vi "诊断标定3.vi"(8 "CAN端口":u16(ring), 9 "设备索引号":u16(ring), 10 "CAN卡类型":u32(ring)=21) -> ()   [LabVIEW 2013] (continued)
                      tunnel: [_ u8 128 ("命令") u8 129 ("命令") u8 128 ("命令") u8 140 ("命令") u8 128 ("命令") u8 128 ("命令") u8 128 ("命令") u8 128 ("命令") u8 128 ("命令") u8 128 ("命令") u8 128 ("命令") u8 128 ("命令") u8 128 ("命令") u8 128 ("命令") u8 128 ("命令") u8 128 ("命令") u8 128 ("命令") u8 129 ("命令") u8 129 ("命令") u8 130 ("命令") u8 130 ("命令") u8 132 ("命令") u8 132 ("命令") u8 132 ("命令") u8 132 ("命令") u8 132 ("命令")] -> w4352
                      tunnel: [_ string[] ["产品编号", "电压个数", "通道电压数", "电压起始值", "温度个数", "温度起始值", "保险位置", "电池额定实际容量", "SOC", "配置文件版本", "参数修改记录", "车牌号", "SOH"] string[] ["一级故障阀值"] string[] ["产品编号"] string[] ["读二维码"] string[] ["电压个数"] string[] ["通道电压数"] string[] ["电压起始值"] string[] ["温度个数"] string[] ["温度起始值"] string[] ["保险位置"] string[] ["SOC"] string[] ["电池额定实际容量"] string[] ["配置文件版本"] string[] ["参数修改记录"] string[] ["校正时钟"] string[] ["车牌号"] string[] ["SOH"] string[] ["二级故障阀值"] string[] ["三级故障阀值"] string[] ["加热控制参数"] string[] ["充电控制参数"] string[] ["电池信息1"] string[] ["电池包组号"] string[] ["充放电安时"] string[] ["电池充放电次数"] string[] ["电池信息1", "电池包组号", "充放电安时", "电池充放电次数"]] -> w4348
                      frame "假", Default {
                      }
                      frame "项目信息" {
                      }
                      frame "SOC过低", "SOC过高", "SOH过低", "充电电流过高", "单体电压过低", "单体电压过高", "单组电压不均衡", "单组温度不均衡", "放电电流过高", "极柱温度过高", "内阻过大", "温度过低", "温度过高", "一级故障阀值", "整组电压不均衡", "整组温度不均衡", "总电压过低", "总电压过高" {
                      }
                      frame "产品编号" {
                      }
                      frame "二维码" {
                      }
                      frame "电压个数" {
                      }
                      frame "通道电压数" {
                      }
                      frame "电压起始值" {
                      }
                      frame "温度个数" {
                      }
                      frame "温度起始值" {
                      }
                      frame "保险位置" {
                      }
                      frame "SOC" {
                      }
                      frame "电池额定实际容量" {
                      }
                      frame "配置文件版本" {
                      }
                      frame "参数修改记录" {
                      }
                      frame "校正时钟" {
                      }
                      frame "车牌号" {
                      }
                      frame "SOH" {
                      }
                      frame "SOC过低(2)", "SOC过高(2)", "SOH过低(2)", "充电电流过高(2)", "单体电压过低(2)", "单体电压过高(2)", "单组电压不均衡(2)", "单组温度不均衡(2)", "二级故障阀值", "放电电流过高(2)", "极柱温度过高(2)", "内阻过大(2)", "温度过低(2)", "温度过高(2)", "整组电压不均衡(2)", "整组温度不均衡(2)", "总电压过低(2)", "总电压过高(2)" {
                      }
                      frame "SOC过低(3)", "SOC过高(3)", "SOH过低(3)", "充电电流过高(3)", "单体电压过低(3)", "单体电压过高(3)", "单组电压不均衡(3)", "单组温度不均衡(3)", "放电电流过高(3)", "极柱温度过高(3)", "内阻过大(3)", "三级故障阀值", "温度过低(3)", "温度过高(3)", "整组电压不均衡(3)", "整组温度不均衡(3)", "总电压过低(3)", "总电压过高(3)" {
                      }
                      frame "风机关闭温差", "风机关闭温度", "风机开启温差", "风机开启温度", "加热关闭温差", "加热关闭温度", "加热开启温度", "加热控制参数" {
                      }
                      frame "充电控制参数", "电流步长", "最大允许充电电流", "最大允许充电温度", "最大允许单体电压", "最大允许总电压", "最小允许充电电流", "最小允许充电温度", "最小允许单体电压" {
                      }
                      frame "电池信息1" {
                      }
                      frame "电池包组号" {
                      }
                      frame "充放电安时" {
                      }
                      frame "电池充放电次数" {
                      }
                      frame "电池信息" {
                      }
                    }
                  }
                  frame "从板" {
                    n3274 = local read "从板选项"() -> (w4434:string)
                    n3275 = case shown="\"二维码\"" w4434 {
                      tunnel: [_ u8 0 ("命令") u8 10 ("命令") u8 0 ("命令") u8 0 ("命令") u8 0 ("命令") u8 0 ("命令") u8 0 ("命令") u8 0 ("命令") u8 2 ("命令") u8 2 ("命令") u8 2 ("命令") u8 3 ("命令") u8 6 ("命令") u8 6 ("命令") u8 6 ("命令") u8 3 ("命令") u8 3 ("命令") u8 3 ("命令") u8 3 ("命令") u8 3 ("命令") u8 3 ("命令") u8 3 ("命令")] -> w4437
                      tunnel: [_ u8[] [6] u8[] [1] u8[] [6, 1, 2, 3, 4, 5] u8[] [1] u8[] [2] u8[] [3] u8[] [4] u8[] [5] u8[] [1] u8[] [2] u8[] [3] u8[] [1, 2, 3, 4, 5, 6, 7] u8[] [1, 2] u8[] [2] u8[] [1] u8[] [1] u8[] [2] u8[] [3] u8[] [4] u8[] [5] u8[] [6] u8[] [7]] -> w4436
                      tunnel: [_ string[] ["从板号"] string[] ["读二维码"] string[] ["从板号", "电压起始值", "通道电压个数", "保险位置", "温度起始值", "加热控制参数"] string[] ["电压起始值"] string[] ["通道电压节数"] string[] ["保险位置"] string[] ["温度起始值"] string[] ["加热控制参数"] string[] ["一级故障阀值"] string[] ["二级故障阀值"] string[] ["三级故障阀值"] string[] ["电池包信息1", "电池包序号", "充放电安时", "充电次数时间", "SOC", "车牌号", "充电参数"] string[] ["均衡阀值", "充电结束电压"] string[] ["充电结束电压"] string[] ["均衡阀值"] string[] ["电池包信息1"] string[] ["电池包序号"] string[] ["充放电安时"] string[] ["充电次数时间"] string[] ["SOC"] string[] ["车牌号"] string[] ["充电参数"]] -> w4432
                      frame "假", Default {
                      }
                      frame "从板号" {
                      }
                      frame "二维码" {
                      }
                      frame "从板信息" {
                      }
                      frame "电压个数" {
                      }
                      frame "通道电压节数" {
                      }
                      frame "保险位置" {
                      }
                      frame "温度个数" {
                      }
                      frame "风机关闭温差", "风机关闭温度", "风机开启温差", "风机开启温度", "加热关闭温差", "加热关闭温度", "加热开启温度", "加热控制参数" {
                      }
                      frame "SOC过低", "电压不均衡", "电压过低", "电压过高", "温度不均衡", "温度过低", "温度过高", "一级故障阀值" {
                      }
                      frame "SOC过低(2)", "电压不均衡(2)", "电压过低(2)", "电压过高(2)", "二级故障阀值", "温度不均衡(2)", "温度过低(2)", "温度过高(2)" {
                      }
                      frame "SOC过低(3)", "电压不均衡(3)", "电压过低(3)", "电压过高(3)", "三级故障阀值", "温度不均衡(3)", "温度过低(3)", "温度过高(3)" {
                      }
                      frame "快换参数" {
                      }
                      frame "均衡参数" {
                      }
                      frame "充电结束电压" {
                      }
                      frame "均衡阀值" {
                      }
                      frame "电池包信息1" {
                      }
                      frame "电池包序号" {
                      }
                      frame "充放电安时" {
                      }
                      frame "充电次数时间" {
                      }
                      frame "SOC" {
                      }
                      frame "车牌号" {
                      }
                      frame "充电参数" {
                      }
                    }
                    n3276 = local read "从板号"() -> (w4433:u8)
                  }
                }
                n3277 = Build Array(w4345) -> (w4344:i32[])
                n3278 = local write "命令"(w4347) -> ()
                n3279 = Array Size(array=w4342) -> (size(s)=w4341:i32)
                n3280 = for {
                  tunnel: w4342 -> [w4512] mode=indexing
                  tunnel: w4347 -> [w4511]
                  tunnel: w4346 -> [w4510]
                  tunnel: w4344 -> [w4509]
                  tunnel: w4343 -> [w4508] mode=indexing
                  tunnel: w4341 -> [w4507]
                  tunnel: w4340 -> [w4505]
                  tunnel: [w4504] -> w4339
                  i -> [w4506]
                  n3281 = while {
                    tunnel: w4512 -> [w4521]
                    tunnel: w4511 -> [w4520]
                    tunnel: w4510 -> [w4519]
                    tunnel: w4509 -> [w4518]
                    tunnel: w4508 -> [w4517]
                    tunnel: w4507 -> [w4516]
                    tunnel: w4506 -> [w4515]
                    tunnel: w4505 -> [w4514]
                    tunnel: [w4513] -> w4504
                    stop <- w4513 stop-if-true
                    n3282 = stacked-sequence {
                      seq-local: [_ _ _ _ w4671 _ _] -> [_ _ _ _ _ w4680 _]
                      tunnel: w4521 -> [_ _ _ w4659 _ _ _]
                      tunnel: w4520 -> [_ _ _ w4658 _ _ _]
                      tunnel: w4519 -> [_ _ _ w4657 _ _ _]
                      tunnel: w4518 -> [_ _ _ w4656 _ _ _]
                      tunnel: [_ _ _ _ w4672 _ _] -> w4513
                      tunnel: w4517 -> [w4523 _ _ _ _ w4681 _]
                      tunnel: w4516 -> [_ _ _ _ _ _ w4691]
                      tunnel: w4515 -> [_ _ _ _ _ _ w4690]
                      tunnel: w4514 -> [w4522 _ _ _ _ _ _]
                      frame #0 {
                        n3283 = case shown="\"从板\"" w4522 {
                          tunnel: w4523 -> [w4524 w4616]
                          frame "主板", Default {
                            n3284 = case shown="\"读二维码\"" w4524 {
                              frame "假", Default {
                              }
                              frame "产品编号" {
                                n3285 = control-ref of="产品编号"() -> (w4526:refnum<vi>)
                                n3286 = property class="Str"(reference=w4526, "Value"="") -> ()  [unwired: 1 in, 2 out]
                              }
                              frame "读二维码" {
                                n3287 = local write "二维码信息"("" ("二维码信息")) -> ()
                              }
                              frame "电压个数" {
                                n3288 = local read "从板个数"() -> (w4528:dbl)
                                n3289 = control-ref of="项目信息"() -> (w4532:refnum<vi>)
                                n3290 = for {
                                N: w4528 -> [_]
                                tunnel: [""] -> w4531 mode=indexing
                                }
                                n3291 = call "表格数据输入-8.6.vi"("行数"=u32 0, "列数"=u32 1, "字符串数组"=w4531, "表格引用"=w4532) -> ()  [unwired: 8 in]
                              }
                              frame "通道电压数" {
                                n3292 = control-ref of="项目信息"() -> (w4538:refnum<vi>)
                                n3293 = for {
                                N: 20 -> [_]
                                tunnel: [""] -> w4537 mode=indexing
                                }
                                n3294 = local read "从板个数"() -> (w4539:dbl)
                                n3295 = Increment(x=w4539) -> (x+1=w4535:dbl)
                                n3296 = call "表格数据输入-8.6.vi"("行数"=w4535, "列数"=u32 1, "字符串数组"=w4537, "表格引用"=w4538) -> ()  [unwired: 8 in]
                              }
                              frame "电压起始值" {
                                n3297 = local read "从板个数"() -> (w4543:dbl)
                                n3298 = Increment(x=w4543) -> (x+1=w4542:dbl)
                                n3299 = control-ref of="项目信息"() -> (w4549:refnum<vi>)
                                n3300 = for {
                                N: w4542 -> [_]
                                tunnel: [""] -> w4548 mode=indexing
                                }
                                n3301 = Multiply(x=u8 1, y=w4543) -> (x*y=w4545:dbl)
                                n3302 = Add(x=w4545, y=u8 21) -> (x+y=w4541:dbl)
                                n3303 = call "表格数据输入-8.6.vi"("行数"=w4541, "列数"=u32 1, "字符串数组"=w4548, "表格引用"=w4549) -> ()  [unwired: 8 in]
                              }
                              frame "温度个数" {
                                n3304 = local read "从板个数"() -> (w4553:dbl)
                                n3305 = Increment(x=w4553) -> (x+1=w4552:dbl)
                                n3306 = control-ref of="项目信息"() -> (w4559:refnum<vi>)
                                n3307 = for {
                                N: w4552 -> [_]
                                tunnel: [""] -> w4558 mode=indexing
                                }
                                n3308 = Multiply(x=u8 2, y=w4553) -> (x*y=w4555:dbl)
                                n3309 = Add(x=w4555, y=u8 22) -> (x+y=w4551:dbl)
                                n3310 = call "表格数据输入-8.6.vi"("行数"=w4551, "列数"=u32 1, "字符串数组"=w4558, "表格引用"=w4559) -> ()  [unwired: 8 in]
                              }
                              frame "温度起始值" {
                                n3311 = local read "从板个数"() -> (w4563:dbl)
                                n3312 = Increment(x=w4563) -> (x+1=w4562:dbl)
                                n3313 = control-ref of="项目信息"() -> (w4569:refnum<vi>)
                                n3314 = for {
                                N: w4562 -> [_]
                                tunnel: [""] -> w4568 mode=indexing
                                }
                                n3315 = Multiply(x=u8 3, y=w4563) -> (x*y=w4565:dbl)
                                n3316 = Add(x=w4565, y=u8 23) -> (x+y=w4561:dbl)
                                n3317 = call "表格数据输入-8.6.vi"("行数"=w4561, "列数"=u32 1, "字符串数组"=w4568, "表格引用"=w4569) -> ()  [unwired: 8 in]
                              }
                              frame "保险位置" {
                                n3318 = local read "从板个数"() -> (w4573:dbl)
                                n3319 = control-ref of="项目信息"() -> (w4579:refnum<vi>)
                                n3320 = for {
                                N: 10 -> [_]
                                tunnel: [""] -> w4578 mode=indexing
                                }
                                n3321 = Multiply(x=u8 4, y=w4573) -> (x*y=w4575:dbl)
                                n3322 = Add(x=w4575, y=u8 24) -> (x+y=w4572:dbl)
                                n3323 = call "表格数据输入-8.6.vi"("行数"=w4572, "列数"=u32 1, "字符串数组"=w4578, "表格引用"=w4579) -> ()  [unwired: 8 in]
                              }
                              frame "电池额定实际容量" {
                                w4581 = 0.0 ("值")
                                n3324 = control-ref of="电池实际容量(A)"() -> (w4582:refnum<vi>)
                                n3325 = control-ref of="电池额定容量(A)"() -> (w4583:refnum<vi>)
                                n3326 = property class="DigNum (严格)"(reference=w4582, "Value"=w4581) -> ()  [unwired: 1 in, 2 out]
                                n3327 = property class="DigNum (严格)"(reference=w4583, "Value"=w4581) -> ()  [unwired: 1 in, 2 out]
                              }
                              frame "SOC" {
                                n3328 = control-ref of="SOC(%)"() -> (w4584:refnum<vi>)
                                n3329 = property class="DigNum (严格)"(reference=w4584, "Value"=0.0 ("值")) -> ()  [unwired: 1 in, 2 out]
                              }
                              frame "配置文件版本" {
                                n3330 = control-ref of="配置文件版本"() -> (w4586:refnum<vi>)
                                n3331 = property class="Str"(reference=w4586, "Value"="" ("值")) -> ()  [unwired: 1 in, 2 out]
                              }
                              frame "参数修改记录" {
                                n3332 = control-ref of="使用者"() -> (w4589:refnum<vi>)
                                n3333 = control-ref of="系统时钟"() -> (w4590:refnum<vi>)
                                n3334 = property class="DigNum (严格)"(reference=w4589, "Value"=0.0 ("值")) -> ()  [unwired: 1 in, 2 out]
                                n3335 = property class="Str"(reference=w4590, "Value"="" ("值")) -> ()  [unwired: 1 in, 2 out]
                              }
                              frame "校正时钟" {
                                n3336 = control-ref of="系统时钟"() -> (w4592:refnum<vi>)
                                n3337 = property class="Str"(reference=w4592, "Value"="" ("值")) -> ()  [unwired: 1 in, 2 out]
                              }
                              frame "车牌号" {
                                n3338 = control-ref of="车架(牌)号"() -> (w4594:refnum<vi>)
                                n3339 = property class="Str"(reference=w4594, "Value"="" ("值")) -> ()  [unwired: 1 in, 2 out]
                              }
                              frame "SOH" {
                                n3340 = control-ref of="SOH(%)"() -> (w4597:refnum<vi>)
                                n3341 = property class="DigNum (严格)"(reference=w4597, "Value"=0.0 ("值")) -> ()  [unwired: 1 in, 2 out]
                              }
                              frame "一级故障阀值" {
                                n3342 = local write "一级故障"(T10 {"总电压过高"=0.0, "整组电压不均衡"=0.0, "SOC过高"=0.0, "单体电压过高"=0.0, "总电压过低"=0.0, "温度过高"=0.0, "温度过低"=0.0, "单组电压不均衡"=0.0, "整组温度不均衡"=0.0, "单组温度不均衡"=0.0, "单体电压过低"=0.0, "充电电流过高"=0.0, "放电电流过高"=0.0, "SOC过低"=0.0, "内阻过大"=0.0, "极柱温度过高"=0.0, "SOH过低"=0.0} ("一级故障")) -> ()
                              }
                              frame "二级故障阀值" {
                                n3343 = local write "一级故障 2"(T10 {"总电压过高"=0.0, "整组电压不均衡"=0.0, "SOC过高"=0.0, "单体电压过高"=0.0, "总电压过低"=0.0, "温度过高"=0.0, "温度过低"=0.0, "单组电压不均衡"=0.0, "整组温度不均衡"=0.0, "单组温度不均衡"=0.0, "单体电压过低"=0.0, "充电电流过高"=0.0, "放电电流过高"=0.0, "SOC过低"=0.0, "内阻过大"=0.0, "极柱温度过高"=0.0, "SOH过低"=0.0} ("一级故障")) -> ()
                              }
                              frame "三级故障阀值" {
                                n3344 = local write "一级故障 3"(T10 {"总电压过高"=0.0, "整组电压不均衡"=0.0, "SOC过高"=0.0, "单体电压过高"=0.0, "总电压过低"=0.0, "温度过高"=0.0, "温度过低"=0.0, "单组电压不均衡"=0.0, "整组温度不均衡"=0.0, "单组温度不均衡"=0.0, "单体电压过低"=0.0, "充电电流过高"=0.0, "放电电流过高"=0.0, "SOC过低"=0.0, "内阻过大"=0.0, "极柱温度过高"=0.0, "SOH过低"=0.0} ("一级故障")) -> ()
                              }
                              frame "加热控制参数" {
                                n3345 = local write "加热控制参数"(T11 {"风机开启温度"=0.0, "风机关闭温度"=0.0, "加热开启温度"=0.0, "加热关闭温度"=0.0, "风机开启温差"=0.0, "风机关闭温差"=0.0, "加热关闭温差"=0.0} ("加热控制参数")) -> ()
                              }
                              frame "充电控制参数" {
                                n3346 = local write "一级故障 5"(T12 {"最大允许单体电压"=0.0, "最大允许总电压"=0.0, "最小允许单体电压"=0.0, "最大允许充电电流"=0.0, "最小允许充电电流"=0.0, "最大允许充电温度"=0.0, "最小允许充电温度"=0.0, "电流步长"=0.0} ("一级故障 5")) -> ()
                              }
                              frame "电池信息1" {
                                w4603 = ""
                                w4604 = 0.0 ("电池串联")
                                n3347 = local read "电池信息"() -> (w4606:T13)
                                n3348 = Bundle By Name(cluster=w4606, "电池串联"=w4604, "电池并联"=w4604, "电池包额定容量"=w4604, "电池包额定能量(kWh)"=w4604, "电池包额定总电压"=w4604, "实际容量"=w4604, "电池厂家"=w4603, "电池类型"=w4603, "电池生产日期"=w4603) -> (w4605:T13)
                                n3349 = local write "电池信息"(w4605) -> ()
                              }
                              frame "电池包组号" {
                                n3350 = local read "电池信息"() -> (w4609:T13)
                                n3351 = Bundle By Name(cluster=w4609, "电池包组号"="") -> (w4608:T13)
                                n3352 = local write "电池信息"(w4608) -> ()
                              }
                              frame "充放电安时" {
                                w4610 = 0.0 ("累计充电总安时")
                                n3353 = local read "电池信息"() -> (w4612:T13)
                                n3354 = Bundle By Name(cluster=w4612, "累计充电总安时"=w4610, "累计放电总安时"=w4610) -> (w4611:T13)
                                n3355 = local write "电池信息"(w4611) -> ()
                              }
                              frame "电池充放电次数" {
                                w4613 = 0.0 ("累计充电总安时")
                                n3356 = local read "电池信息"() -> (w4615:T13)
                                n3357 = Bundle By Name(cluster=w4615, "电池充满次数"=w4613, "电池放空次数"=w4613, "电池充电次数"=w4613) -> (w4614:T13)
                                n3358 = local write "电池信息"(w4614) -> ()
                              }
                            }
                          }
                          frame "从板" {
                            n3359 = case shown="\"读二维码\"" w4616 {
                              frame "假", Default {
                              }
                              frame "电压起始值" {
                                n3360 = control-ref of="项目信息 2"() -> (w4618:refnum<vi>)
                                n3361 = for {
                                N: 1 -> [_]
                                tunnel: [""] -> w4621 mode=indexing
                                }
                                n3362 = call "表格数据输入-8.6.vi"("行数"=u32 0, "列数"=u32 1, "字符串数组"=w4621, "表格引用"=w4618) -> ()  [unwired: 8 in]
                              }
                              frame "读二维码" {
                                n3363 = local write "二维码信息 2"("" ("二维码信息 2")) -> ()
                              }
                              frame "通道电压节数" {
                                n3364 = control-ref of="项目信息 2"() -> (w4624:refnum<vi>)
                                n3365 = for {
                                N: 5 -> [_]
                                tunnel: [""] -> w4628 mode=indexing
                                }
                                n3366 = call "表格数据输入-8.6.vi"("行数"=u32 22, "列数"=u32 1, "字符串数组"=w4628, "表格引用"=w4624) -> ()  [unwired: 8 in]
                              }
                              frame "保险位置" {
                                n3367 = control-ref of="项目信息 2"() -> (w4630:refnum<vi>)
                                n3368 = for {
                                N: 20 -> [_]
                                tunnel: [""] -> w4634 mode=indexing
                                }
                                n3369 = call "表格数据输入-8.6.vi"("行数"=u32 2, "列数"=u32 1, "字符串数组"=w4634, "表格引用"=w4630) -> ()  [unwired: 8 in]
                              }
                              frame "温度起始值" {
                                n3370 = control-ref of="项目信息 2"() -> (w4636:refnum<vi>)
                                n3371 = for {
                                N: 1 -> [_]
                                tunnel: [""] -> w4640 mode=indexing
                                }
                                n3372 = call "表格数据输入-8.6.vi"("行数"=u32 1, "列数"=u32 1, "字符串数组"=w4640, "表格引用"=w4636) -> ()  [unwired: 8 in]
                              }
                              frame "加热控制参数" {
                                n3373 = local write "加热控制参数"(T11 {"风机开启温度"=0.0, "风机关闭温度"=0.0, "加热开启温度"=0.0, "加热关闭温度"=0.0, "风机开启温差"=0.0, "风机关闭温差"=0.0, "加热关闭温差"=0.0} ("加热控制参数")) -> ()
                              }
                              frame "一级故障阀值" {
                                n3374 = local write "一级故障 6"(T15 {"电压过高"=0.0, "电压过低"=0.0, "温度过高"=0.0, "温度过低"=0.0, "电压不均衡(V)"=0.0, "温度不均衡"=0.0, "SOC过低"=0.0} ("一级故障 6")) -> ()
                              }
                              frame "二级故障阀值" {
                                n3375 = local write "一级故障 7"(T15 {"电压过高"=0.0, "电压过低"=0.0, "温度过高"=0.0, "温度过低"=0.0, "电压不均衡(V)"=0.0, "温度不均衡"=0.0, "SOC过低"=0.0} ("一级故障 7")) -> ()
                              }
                              frame "三级故障阀值" {
                                n3376 = local write "一级故障 8"(T15 {"电压过高"=0.0, "电压过低"=0.0, "温度过高"=0.0, "温度过低"=0.0, "电压不均衡(V)"=0.0, "温度不均衡"=0.0, "SOC过低"=0.0} ("一级故障 7")) -> ()
                              }
                              frame "均衡参数" {
                                n3377 = local write "均衡参数"(T17 {"充电结束电压(90%)"=0.0, "充电结束电压(91%)"=0.0, "充电结束电压(92%)"=0.0, "充电结束电压(93%)"=0.0, "充电结束电压(94%)"=0.0, "均衡计算-电压高阀值1级"=0.0, "均衡计算-电压高阀值2级"=0.0, "均衡计算-电压低阀值1级"=0.0, "均衡计算-电压低阀值2级"=0.0, "均衡计算-最低电压阀值"=0.0, "均衡停止-最低电压阀值"=0.0, "均衡计算-电压极差阀值"=0.0, "充电结束电压(95%)"=0.0, "充电结束电压(96%)"=0.0, "充电结束电压(97%)"=0.0, "充电结束电压(98%)"=0.0, "充电结束电压(99%)"=0.0, "充电结束电压(100%)"=0.0} ("均衡参数")) -> ()
                              }
                              frame "均衡阀值" {
                                w4647 = sgl 0.0 ("均衡计算-电压高阀值1级")
                                n3378 = local read "均衡参数"() -> (w4648:T17)
                                n3379 = Bundle By Name(cluster=w4648, "均衡计算-电压高阀值1级"=w4647, "均衡计算-电压高阀值2级"=w4647, "均衡计算-电压低阀值1级"=w4647, "均衡计算-电压低阀值2级"=w4647, "均衡计算-最低电压阀值"=w4647, "均衡停止-最低电压阀值"=w4647, "均衡计算-电压极差阀值"=w4647) -> (w4649:T17)
                                n3380 = local write "均衡参数"(w4649) -> ()
                              }
                              frame "充电结束电压" {
                                w4650 = sgl 0.0 ("均衡计算-电压高阀值1级")
                                n3381 = local read "均衡参数"() -> (w4651:T17)
                                n3382 = Bundle By Name(cluster=w4651, "充电结束电压(90%)"=w4650, "充电结束电压(91%)"=w4650, "充电结束电压(92%)"=w4650, "充电结束电压(93%)"=w4650, "充电结束电压(94%)"=w4650, "充电结束电压(95%)"=w4650, "充电结束电压(96%)"=w4650, "充电结束电压(97%)"=w4650, "充电结束电压(98%)"=w4650, "充电结束电压(99%)"=w4650, "充电结束电压(100%)"=w4650) -> (w4652:T17)
                                n3383 = local write "均衡参数"(w4652) -> ()
                              }
                            }
                          }
                        }
                      }
                      frame #1 {
                        w4653 = FALSE ("流控帧")
                        w4654 = TRUE ("流控帧 2")
                        n3384 = global write "EV05全局变量1.vi" "写入超时"(w4653) -> ()
                        n3385 = global write "EV05全局变量1.vi" "流控帧"(w4653) -> ()
                        n3386 = local write "写?"(w4653) -> ()
                        n3387 = call <vilib>:"Set Busy.vi"("disable click? (T)"=w4653) -> ()  [unwired: 3 in, 8 out]
                        n3388 = local write "消除"(w4654) -> ()
                        n3389 = local write "控制1"(w4654) -> ()
                        n3390 = global write "EV05全局变量1.vi" "流控帧 2"(w4654) -> ()
                      }
                      frame #2 {
                        n3391 = Wait Until Next ms Multiple(millisecond multiple=u32 150 ("毫秒倍数")) -> ()  [unwired: 1 out]
                      }
                      frame #3 {
                        n3392 = local read "设备索引号"() -> (w4661:u16)
                        n3393 = local read "CAN卡类型"() -> (w4662:u32)
                        n3394 = local read "CAN端口"() -> (w4660:u16)
                        n3395 = stacked-sequence {
                          tunnel: w4662 -> [_ w4670]
                          tunnel: w4661 -> [_ w4669]
                          tunnel: w4660 -> [_ w4668]
                          tunnel: w4659 -> [_ w4667]
                          tunnel: w4658 -> [_ w4666]
                          tunnel: w4657 -> [_ w4665]
                          tunnel: w4656 -> [_ w4664]
                          frame #0 {
                          }
                          frame #1 {
                            n3396 = call "多帧发送机制(EV05).vi"("can卡类型"=w4670, "设备索引号"=w4669, "CAN端口"=w4668, "命令"=w4666, "板号"=w4665, "命令序号"=w4667, "输入数据"=w4664) -> ("错误输出"=w4663:errorcluster)  [unwired: 1 in, 11 out]
                            n3397 = call <vilib>:"Clear Errors.vi"("error in (no error)"=w4663) -> ()  [unwired: 6 in, 1 out]
                          }
                        }
                        "命令序号" <- w4659
                      }
                      frame #4 {
                        n3398 = while {
                          tunnel: [w4675] -> w4672
                          tunnel: [w4674] -> w4671
                          i -> [w4678]
                          stop <- w4675 stop-if-true
                          n3399 = local read "强制终止读写标记"() -> (w4673:bool)
                          n3400 = global read "EV05全局变量1.vi" "写入超时"() -> (w4674:bool)
                          n3401 = Greater Or Equal?(x=w4678, y=30) -> (x >= y?=w4676:bool)
                          n3402 = Compound Arithmetic op=OR(w4673, w4674, w4676) -> (w4675:bool)
                          n3403 = Wait Until Next ms Multiple(millisecond multiple=u32 100 ("毫秒倍数")) -> ()  [unwired: 1 out]
                        }
                      }
                      frame #5 {
                        n3404 = case shown="假" w4680 {
                          tunnel: w4681 -> [w4684 _]
                          frame False {
                            n3405 = control-ref of="结果"() -> (w4683:refnum<vi>)
                            n3406 = Concatenate Strings(w4684, "     读取失败" ("字符串")) -> (w4686:string)
                            n3407 = Build Array(w4686) -> (w4682:string[])
                            n3408 = call "表格编辑.vi"("新元素/子数组"=w4682, "活动单元格:单元格背景色"=u32 16740749, "MCListbox引用句柄"=w4683) -> ()  [unwired: 9 out]
                          }
                          frame True {
                          }
                        }
                      }
                      frame #6 {
                        n3409 = Increment(x=w4690) -> (x+1=w4689:i32)
                        n3410 = Equal?(x=w4691, y=w4689) -> (x = y?=w4688:bool)
                        n3411 = case shown="真" w4688 {
                          frame False {
                          }
                          frame True {
                            n3412 = control-ref of="结果"() -> (w4693:refnum<vi>)
                            n3413 = Concatenate Strings("读取完成" ("字符串")) -> (w4695:string)
                            n3414 = Build Array(w4695) -> (w4692:string[])
                            n3415 = call "表格编辑.vi"("新元素/子数组"=w4692, "活动单元格:单元格背景色"=u32 21937, "MCListbox引用句柄"=w4693) -> ()  [unwired: 9 out]
                          }
                        }
                      }
                    }
                  }
                }
              }
            }
            n3416 = stacked-sequence {
              tunnel: w4337 -> [_]
              frame #0 {
                n3417 = call <vilib>:"Unset Busy.vi"() -> ()  [unwired: 11 in, 1 out]
                n3418 = local write "强制终止读写标记"(FALSE ("强制停止")) -> ()
              }
            }
          }
          frame "全部读取" {
            n3419 = stacked-sequence {
              seq-local: [w4701 _ _] -> [_ _ w5262]
              seq-local: [w4700 _ _] -> [_ _ w5261]
              tunnel: [_ w4892 _] -> w4698
              frame #0 {
                n3420 = local read "主从选择"() -> (w4701:enum32{"主板", "从板"})
                n3421 = local read "路径"() -> (w4702:path)
                n3422 = Empty String/Path?(string/path=w4702) -> (empty?=w4700:bool)
                n3423 = disable-structure shown="禁用" {
                  disable-tunnel: w4702 -> [w4705 _]
                  disable-tunnel: w4700 -> [w4704 _]
                  disable-tunnel: w4701 -> [w4703 _]
                  frame Disabled {
                    n3424 = case shown="假" w4704 {
                      tunnel: w4705 -> [w4709 _]
                      tunnel: w4703 -> [w4708 _]
                      frame False {
                        n3425 = control-ref of="结果"() -> (w4706:refnum<vi>)
                        n3426 = call-poly <vilib>:"Read From Spreadsheet File.vi"("file path (dialog if empty)"=w4709) -> ("all rows"=w4707:string[][])  [unwired: 3 in, 7 out]
                        n3427 = case shown="\"主板\", 默认" w4708 {
                          tunnel: w4707 -> [w4711 w4806]
                          tunnel: w4706 -> [w4710 w4805]
                          frame "主板", Default {
                            n3428 = stacked-sequence {
                              tunnel: w4711 -> [w4720 w4744 w4801]
                              tunnel: w4710 -> [w4717 _ w4772]
                              frame #0 {
                                n3429 = Index Array(array=w4720, index (col)=3 ("禁用的索引 (列)")) -> (element=w4734:string[])  [unwired: 1 in]
                                n3430 = Index Array(array=w4720, index (col)=1 ("禁用的索引 (列)")) -> (element=w4740:string[])  [unwired: 1 in]
                                n3431 = Delete From Array(array=w4734, length=4 ("长度"), index=0 ("索引")) -> (deleted portion=w4731:string[], array with subset deleted=w4725:string[])
                                n3432 = Delete From Array(array=w4740, length=1 ("长度"), index=0 ("索引")) -> (deleted portion=w4737:string[], array with subset deleted=w4714:string[])
                                n3433 = Build Array("正在读取主板配置文件...") -> (w4718:string[])
                                n3434 = Index Array(array=w4725) -> (element #1=w4724:string, element #2=w4723:string, element #3=w4722:string, element #4=w4721:string)  [unwired: 4 in]
                                n3435 = for {
                                tunnel: w4731 -> [w4743] mode=indexing
                                tunnel: [w4742] -> w4730 mode=indexing
                                n3436 = Fract/Exp String To Number(string=w4743) -> (number=w4742:dbl)  [unwired: 4 out]
                                }
                                n3437 = Index Array(array=w4737) -> (element=w4736:string)  [unwired: 1 in]
                                n3438 = global write "读配置文件全局.vi" "表格输入"(w4714) -> ()
                                n3439 = call "表格编辑.vi"("新元素/子数组"=w4718, "活动单元格:单元格背景色"=u32 6618880, "MCListbox引用句柄"=w4717) -> ()  [unwired: 9 out]
                                n3440 = Decimal String To Number(string=w4736) -> (number=w4715:i32)  [unwired: 1 in, 2 out]
                                n3441 = global read "读配置文件全局.vi" "项目信息"() -> (w4713:T27)
                                n3442 = Index Array(array=w4730) -> (element #1=w4729:dbl, element #2=w4728:dbl, element #3=w4727:dbl, element #4=w4726:dbl)  [unwired: 4 in]
                                n3443 = global write "读配置文件全局.vi" "从板个数"(w4715) -> ()
                                n3444 = Bundle(cluster=w4713, "电池额定容量"=w4729, "电池实际容量"=w4728, "车牌号"=w4724, "配置文件版本"=w4723, "SOH"=w4726, "SOC"=w4727, "产品编号"=w4722, "系统时钟"=w4721) -> (w4712:T27)  [unwired: 1 out]
                                n3445 = global write "读配置文件全局.vi" "项目信息"(w4712) -> ()
                              }
                              frame #1 {
                                n3446 = Index Array(array=w4744, index (col)=3 ("禁用的索引 (列)")) -> (element=w4762:string[])  [unwired: 1 in]
                                n3447 = Index Array(array=w4744, index (col)=5 ("禁用的索引 (列)")) -> (element=w4756:string[])  [unwired: 1 in]
                                n3448 = for {
                                tunnel: w4756 -> [w4769] mode=indexing
                                tunnel: [w4768] -> w4755 mode=indexing
                                n3449 = Fract/Exp String To Number(string=w4769) -> (number=w4768:dbl)  [unwired: 4 out]
                                }
                                n3450 = Delete From Array(array=w4762, length=17 ("长度"), index=8 ("索引")) -> (deleted portion=w4760:string[])  [unwired: 1 out]
                                n3451 = for {
                                tunnel: w4760 -> [w4771] mode=indexing
                                tunnel: [w4770] -> w4758 mode=indexing
                                n3452 = Fract/Exp String To Number(string=w4771) -> (number=w4770:dbl)  [unwired: 4 out]
                                }
                                n3453 = global write "读配置文件全局.vi" "二级故障"(w4755) -> ()
                                n3454 = global write "读配置文件全局.vi" "一级故障"(w4758) -> ()
                                n3455 = Index Array(array=w4744, index (col)=7 ("禁用的索引 (列)")) -> (element=w4753:string[])  [unwired: 1 in]
                                n3456 = Index Array(array=w4744, index (col)=9 ("禁用的索引 (列)")) -> (element=w4750:string[])  [unwired: 1 in]
                                n3457 = for {
                                tunnel: w4753 -> [w4767] mode=indexing
                                tunnel: [w4766] -> w4752 mode=indexing
                                n3458 = Fract/Exp String To Number(string=w4767) -> (number=w4766:dbl)  [unwired: 4 out]
                                }
                                n3459 = for {
                                tunnel: w4750 -> [w4765] mode=indexing
                                tunnel: [w4764] -> w4749 mode=indexing
                                n3460 = Fract/Exp String To Number(string=w4765) -> (number=w4764:dbl)  [unwired: 4 out]
                                }
                                n3461 = Delete From Array(array=w4749, length=6 ("长度"), index=0 ("索引")) -> (deleted portion=w4746:dbl[], array with subset deleted=w4745:dbl[])
                                n3462 = global write "读配置文件全局.vi" "三级故障"(w4752) -> ()
                                n3463 = global write "读配置文件全局.vi" "加热控制参数"(w4746) -> ()
                                n3464 = global write "读配置文件全局.vi" "充电控制参数"(w4745) -> ()
                              }
                              frame #2 {
                                n3465 = call <vilib>:"Unset Busy.vi"() -> ()  [unwired: 2 in, 10 out]
                                n3466 = Index Array(array=w4801, index (col)=11 ("禁用的索引 (列)")) -> (element=w4798:string[])  [unwired: 1 in]
                                n3467 = Delete From Array(array=w4798, length=6 ("长度"), index=0 ("索引")) -> (deleted portion=w4780:string[], array with subset deleted=w4779:string[])
                                n3468 = for {
                                tunnel: w4779 -> [w4804] mode=indexing
                                tunnel: [w4803] -> w4797 mode=indexing
                                n3469 = Fract/Exp String To Number(string=w4804) -> (number=w4803:dbl)  [unwired: 4 out]
                                }
                                n3470 = Index Array(array=w4780) -> (element #1=w4796:string, element #2=w4795:string, element #3=w4794:string, element #4=w4793:string, element #5=w4792:string, element #6=w4791:string)  [unwired: 6 in]
                                n3471 = Index Array(array=w4797) -> (element #1=w4790:dbl, element #2=w4789:dbl, element #3=w4788:dbl, element #4=w4787:dbl, element #5=w4786:dbl, element #6=w4785:dbl, element #7=w4784:dbl, element #8=w4783:dbl, element #9=w4782:dbl, element #10=w4781:dbl, element #11=w4776:dbl)  [unwired: 11 in]
                                n3472 = global read "读配置文件全局.vi" "电池信息"() -> (w4778:T28)
                                n3473 = Build Array("配置文件读取完成") -> (w4774:string[])
                                n3474 = Bundle(cluster=w4778, "电池串联"=w4790, "电池并联"=w4789, "累计放电总安时"=w4787, "电池包额定容量"=w4786, "电池包额定能量"=w4785, "电池包额定总电压"=w4784, "累计充电总安时"=w4788, "电池充满次数"=w4783, "电池放空次数"=w4782, "电池充电次数"=w4781, "电池生产日期"=w4796, "电池厂家"=w4795, "电池类型"=w4794, "电池包组号"=w4793, "电池包产权标识"=w4792, "电池应用车型"=w4791, "实际容量"=w4776) -> (w4777:T28)
                                n3475 = call "表格编辑.vi"("新元素/子数组"=w4774, "活动单元格:单元格背景色"=u32 6618880, "MCListbox引用句柄"=w4772) -> ()  [unwired: 9 out]
                                n3476 = global write "读配置文件全局.vi" "电池信息"(w4777) -> ()
                              }
                            }
                          }
                          frame "从板" {
                            n3477 = stacked-sequence {
                              tunnel: w4806 -> [w4814 w4842 w4886]
                              tunnel: w4805 -> [w4811 _ w4862]
                              frame #0 {
                                n3478 = Index Array(array=w4814, index (col)=1 ("禁用的索引 (列)")) -> (element=w4824:string[])  [unwired: 1 in]
                                n3479 = Index Array(array=w4814, index (col)=3 ("禁用的索引 (列)")) -> (element=w4818:string[])  [unwired: 1 in]
                                n3480 = Delete From Array(array=w4824, length=1 ("长度"), index=0 ("索引")) -> (deleted portion=w4821:string[], array with subset deleted=w4808:string[])
                                n3481 = Delete From Array(array=w4818, length=6 ("长度"), index=0 ("索引")) -> (deleted portion=w4815:string[])  [unwired: 1 out]
                                n3482 = for {
                                tunnel: w4815 -> [w4827] mode=indexing
                                tunnel: [w4826] -> w4807 mode=indexing
                                i -> [w4828]
                                n3483 = Fract/Exp String To Number(string=w4827, default (0 dbl)=w4828) -> (number=w4826:i32)  [unwired: 3 out]
                                }
                                n3484 = Index Array(array=w4821) -> (element=w4820:string)  [unwired: 1 in]
                                n3485 = global write "读配置文件全局2.vi" "表格"(w4808) -> ()
                                n3486 = Build Array("正在读取从板配置文件...") -> (w4812:string[])
                                n3487 = Decimal String To Number(string=w4820) -> (number=w4809:i32)  [unwired: 1 in, 2 out]
                                n3488 = call "表格编辑.vi"("新元素/子数组"=w4812, "活动单元格:单元格背景色"=u32 6618880, "MCListbox引用句柄"=w4811) -> ()  [unwired: 9 out]
                                n3489 = global write "读配置文件全局2.vi" "加热控制参数"(w4807) -> ()
                                n3490 = global write "读配置文件全局2.vi" "从板板号"(w4809) -> ()
                              }
                              frame #1 {
                                n3491 = Index Array(array=w4842, index (col)=3 ("禁用的索引 (列)")) -> (element=w4832:string[])  [unwired: 1 in]
                                n3492 = Array Subset(array=w4832, index=6 ("索引"), length=7 ("长度")) -> (w4839:string[])
                                n3493 = Array Subset(array=w4832, index=13 ("索引"), length=7 ("长度")) -> (w4838:string[])
                                n3494 = Array Subset(array=w4832, index=20 ("索引"), length=7 ("长度")) -> (w4833:string[])
                                n3495 = for {
                                tunnel: w4839 -> [w4849] mode=indexing
                                tunnel: [w4848] -> w4829 mode=indexing
                                n3496 = Fract/Exp String To Number(string=w4849) -> (number=w4848:dbl)  [unwired: 4 out]
                                }
                                n3497 = for {
                                tunnel: w4838 -> [w4847] mode=indexing
                                tunnel: [w4846] -> w4830 mode=indexing
                                n3498 = Fract/Exp String To Number(string=w4847) -> (number=w4846:dbl)  [unwired: 4 out]
                                }
                                n3499 = for {
                                tunnel: w4833 -> [w4845] mode=indexing
                                tunnel: [w4844] -> w4831 mode=indexing
                                n3500 = Fract/Exp String To Number(string=w4845) -> (number=w4844:dbl)  [unwired: 4 out]
                                }
                                n3501 = global write "读配置文件全局2.vi" "一级故障阀值"(w4829) -> ()
                                n3502 = global write "读配置文件全局2.vi" "二级故障阀值"(w4830) -> ()
                                n3503 = global write "读配置文件全局2.vi" "三级故障阀值"(w4831) -> ()
                              }
                              frame #2 {
                                n3504 = Index Array(array=w4886, index (col)=5 ("禁用的索引 (列)")) -> (element=w4884:string[])  [unwired: 1 in]
                                n3505 = Delete From Array(array=w4884, length=1 ("长度"), index=16 ("索引")) -> (deleted portion=w4880:string[], array with subset deleted=w4881:string[])
                                n3506 = for {
                                tunnel: w4881 -> [w4889] mode=indexing
                                tunnel: [w4888] -> w4885 mode=indexing
                                n3507 = Fract/Exp String To Number(string=w4889) -> (number=w4888:dbl)  [unwired: 4 out]
                                }
                                n3508 = Index Array(array=w4885) -> (element #1=w4879:dbl, element #2=w4878:dbl, element #3=w4877:dbl, element #4=w4876:dbl, element #5=w4875:dbl, element #6=w4874:dbl, element #7=w4873:dbl, element #8=w4872:dbl, element #9=w4871:dbl, element #10=w4870:dbl, element #11=w4869:dbl, element #12=w4860:dbl, element #13=w4868:dbl, element #14=w4867:dbl, element #15=w4866:dbl, element #16=w4865:dbl, element #17=w4858:dbl, element #18=w4857:dbl, element #19=w4856:dbl, element #20=w4855:dbl, element #21=w4854:dbl, element #22=w4853:dbl)  [unwired: 22 in]
                                n3509 = Build Array("配置文件读取完成") -> (w4863:string[])
                                n3510 = Index Array(array=w4880, index=22 ("索引")) -> (element=w4859:string)
                                n3511 = global read "读配置文件全局2.vi" "电池组信息"() -> (w4851:T29)
                                n3512 = call "表格编辑.vi"("新元素/子数组"=w4863, "活动单元格:单元格背景色"=u32 6618880, "MCListbox引用句柄"=w4862) -> ()  [unwired: 9 out]
                                n3513 = Bundle(cluster=w4851, "电池类型"=w4879, "电池厂家"=w4878, "电池地区"=w4877, "电池组序号"=w4876, "电池包串联数"=w4875, "电池包并联数"=w4874, "电池包安时数"=w4873, "电池包序号"=w4872, "充电次数"=w4871, "充满电时间"=w4870, "放空时间"=w4869, "车牌号"=w4859, "最大允许单体电压"=w4860, "最大允许总电压"=w4868, "最大允许温度"=w4867, "最小允许温度"=w4866, "最大允许充电电流"=w4865, "最小允许充电电流"=w4858, "最小允许单体电压"=w4857, "电流步长"=w4856, "SOC"=w4855, "充电总安时"=w4854, "放电总这时"=w4853) -> (w4850:T29)
                                n3514 = call <vilib>:"Unset Busy.vi"() -> ()  [unwired: 2 in, 10 out]
                                n3515 = global write "读配置文件全局2.vi" "电池组信息"(w4850) -> ()
                              }
                            }
                          }
                        }
                      }
                      frame True {
                      }
                    }
                  }
                  frame Enabled {
                  }
                }
                n3516 = case shown="\"从板\"" w4701 {
                  frame "主板", Default {
                    w4890 = FALSE
                    n3517 = global write "读配置文件全局.vi" "SOC判定"(w4890) -> ()
                    n3518 = global write "读配置文件全局.vi" "SOH判定"(w4890) -> ()
                    n3519 = global write "读配置文件全局.vi" "车牌号判定"(w4890) -> ()
                    n3520 = global write "读配置文件全局.vi" "电池信息1判定"(w4890) -> ()
                    n3521 = global write "读配置文件全局.vi" "保险位置判定"(w4890) -> ()
                    n3522 = global write "读配置文件全局.vi" "产品编号判定"(w4890) -> ()
                    n3523 = global write "读配置文件全局.vi" "充放电安时判定"(w4890) -> ()
                    n3524 = global write "读配置文件全局.vi" "从板个数判定"(w4890) -> ()
                    n3525 = global write "读配置文件全局.vi" "电池包组号判定"(w4890) -> ()
                    n3526 = global write "读配置文件全局.vi" "电压个数判定"(w4890) -> ()
                    n3527 = global write "读配置文件全局.vi" "电压起始值判定"(w4890) -> ()
                    n3528 = global write "读配置文件全局.vi" "二级故障判定"(w4890) -> ()
                    n3529 = global write "读配置文件全局.vi" "三级故障判定"(w4890) -> ()
                    n3530 = global write "读配置文件全局.vi" "通道电压数判定"(w4890) -> ()
                    n3531 = global write "读配置文件全局.vi" "温度个数判定"(w4890) -> ()
                    n3532 = global write "读配置文件全局.vi" "一级故障判定"(w4890) -> ()
                    n3533 = global write "读配置文件全局.vi" "温度起始值判定"(w4890) -> ()
                    n3534 = global write "读配置文件全局.vi" "充电控制参数判定"(w4890) -> ()
                    n3535 = global write "读配置文件全局.vi" "电池充放电次数判定"(w4890) -> ()
                    n3536 = global write "读配置文件全局.vi" "加热控制参数判定"(w4890) -> ()
                    n3537 = global write "读配置文件全局.vi" "配置文件版本判定"(w4890) -> ()
                    n3538 = global write "读配置文件全局.vi" "电池额定实际容量判定"(w4890) -> ()
                  }
                  frame "从板" {
                    w4891 = FALSE
                    n3539 = disable-structure shown="禁用" {
                      frame Disabled {
                        n3540 = global read "读配置文件全局2.vi" "充电次数时间判定"() -> ()  [unwired: 1 in]
                        n3541 = global read "读配置文件全局2.vi" "电池包信息1判定"() -> ()  [unwired: 1 in]
                        n3542 = global read "读配置文件全局2.vi" "电池包序号判定"() -> ()  [unwired: 1 in]
                        n3543 = global read "读配置文件全局2.vi" "充放电安时判定"() -> ()  [unwired: 1 in]
                        n3544 = global read "读配置文件全局2.vi" "车牌号判定"() -> ()  [unwired: 1 in]
                        n3545 = global read "读配置文件全局2.vi" "充电参数判定"() -> ()  [unwired: 1 in]
                        n3546 = global read "读配置文件全局2.vi" "保险位置判定"() -> ()  [unwired: 1 in]
                      }
                      frame Enabled {
                      }
                    }
                    n3547 = global write "读配置文件全局2.vi" "从板号判定"(w4891) -> ()
                    n3548 = global write "读配置文件全局2.vi" "通道电压判定"(w4891) -> ()
                    n3549 = global write "读配置文件全局2.vi" "保险位置判定"(w4891) -> ()
                    n3550 = global write "读配置文件全局2.vi" "二级故障判定"(w4891) -> ()
                    n3551 = global write "读配置文件全局2.vi" "三级故障判定"(w4891) -> ()
                    n3552 = global write "读配置文件全局2.vi" "一级故障判定"(w4891) -> ()
                    n3553 = global write "读配置文件全局2.vi" "电压起始值判定"(w4891) -> ()
                    n3554 = global write "读配置文件全局2.vi" "温度起始值判定"(w4891) -> ()
                  }
                }
              }
              frame #1 {
                (unwired) "均衡参数"
                # "去掉加热控制信息 20140106"
                n3555 = local read "主从选择"() -> (w4895:enum32{"主板", "从板"})
                n3556 = case shown="\"主板\", 默认" w4895 {
                  tunnel: [string[] ["项目信息", "一级故障阀值", "二级故障阀值", "三级故障阀值", "加热控制信息", "充电控制信息", "电池信息", "二维码"] string[] ["从板信息", "一级故障阀值", "二级故障阀值", "三级故障阀值", "二维码"]] -> w4894
                  frame "主板", Default {
                  }
                  frame "从板" {
                  }
                }
                n3557 = Array Size(array=w4894) -> (size(s)=w4893:i32)
                n3558 = for {
                  tunnel: w4894 -> [w4911] mode=indexing
                  tunnel: w4895 -> [w4899]
                  tunnel: w4893 -> [w4903]
                  tunnel: [w4898] -> w4892
                  i -> [w4900]
                  n3559 = case shown="\"主板\", 默认" w4899 {
                    tunnel: [w5207 w5238] -> w4905
                    tunnel: [w5206 w5239] -> w4906
                    tunnel: w4911 -> [w5203 w5235]
                    tunnel: [u8 0 ("板号") w5236] -> w4910
                    tunnel: [u8 0 ("板号") u8 0 ("板号")] -> w4909
                    tunnel: [w5202 w5234] -> w4907
                    frame "主板", Default {
                      n3560 = case shown="\"项目信息\"" w5203 {
                        tunnel: [_ u8[] [1, 2, 3, 4, 5, 6, 13, 8, 7, 9, 10, 11, 12] u8[] [1] u8[] [1] u8[] [2] u8[] [3] u8[] [1] u8[] [2] u8[] [1, 2, 3] u8[] [1, 2, 3, 4]] -> w5207
                        tunnel: [_ u8 128 ("命令") u8 140 ("命令") u8 129 ("命令") u8 129 ("命令") u8 129 ("命令") u8 130 ("命令") u8 130 ("命令") u8 131 ("命令") u8 132 ("命令")] -> w5206
                        tunnel: [_ string[] ["产品编号", "电压个数", "通道电压数", "电压起始值", "温度个数", "温度起始值", "保险位置", "电池额定实际容量", "SOC", "配置文件版本", "参数修改记录", "车牌号", "SOH"] string[] ["读二维码"] string[] ["一级故障阀值"] string[] ["二级故障阀值"] string[] ["三级故障阀值"] string[] ["加热控制参数"] string[] ["充电控制参数"] _ string[] ["电池信息1", "电池包组号", "充放电安时", "电池充放电次数"]] -> w5202
                        frame "假", Default {
                        }
                        frame "项目信息" {
                        }
                        frame "二维码" {
                        }
                        frame "一级故障阀值" {
                        }
                        frame "二级故障阀值" {
                        }
                        frame "三级故障阀值" {
                        }
                        frame "加热控制信息" {
                        }
                        frame "充电控制信息" {
                        }
                        frame "历史信息" {
                        }
                        frame "电池信息" {
                        }
                      }
                    }
                    frame "从板" {
                      n3561 = case shown="\"二维码\"" w5235 {
                        tunnel: [_ u8 0 ("命令") u8 10 ("命令") u8 2 ("命令") u8 2 ("命令") u8 2 ("命令") u8 3 ("命令") u8 6 ("命令")] -> w5239
                        tunnel: [_ u8[] [6, 1, 2, 3, 4, 5] u8[] [1] u8[] [1] u8[] [2] u8[] [3] u8[] [1, 2, 3, 4, 5, 6, 7] u8[] [1, 2]] -> w5238
                        tunnel: [_ string[] ["从板号", "电压起始值", "通道电压节数", "保险位置", "温度起始值", "加热控制参数"] string[] ["读二维码"] string[] ["一级故障阀值"] string[] ["二级故障阀值"] string[] ["三级故障阀值"] string[] ["电池包信息1", "电池包序号", "充放电安时", "充电次数时间", "SOC", "车牌号", "充电参数"] string[] ["均衡阀值", "充电结束电压"]] -> w5234
                        frame "假", Default {
                        }
                        frame "从板信息" {
                        }
                        frame "二维码" {
                        }
                        frame "一级故障阀值" {
                        }
                        frame "二级故障阀值" {
                        }
                        frame "三级故障阀值" {
                        }
                        frame "快换参数" {
                        }
                        frame "均衡参数" {
                        }
                      }
                      n3562 = local read "从板号"() -> (w5236:u8)
                    }
                  }
                  n3563 = Increment(x=w4900) -> (x+1=w4902:i32)
                  n3564 = Equal?(x=w4903, y=w4902) -> (x = y?=w4901:bool)
                  n3565 = case shown="\"从板\"" w4899 {
                    tunnel: w4900 -> [w5173 w5187]
                    frame "主板", Default {
                      n3566 = case shown="0, 默认" w5173 {
                        tunnel: [T8."项目信息" ("主从板") T8."一级故障阀值" ("主从板") T8."二级故障阀值" ("主从板") T8."三级故障阀值" ("主从板") T8."控制参数" ("主从板") T8."电池信息" ("主从板")] -> w5172
                        frame 0, Default {
                          n3567 = local write "1"(TRUE ("1")) -> ()
                        }
                        frame 1 {
                          n3568 = local write "1 2"(TRUE ("1 2")) -> ()
                        }
                        frame 2 {
                          n3569 = local write "1 3"(TRUE ("1 3")) -> ()
                        }
                        frame 3 {
                          n3570 = local write "1 4"(TRUE ("1 4")) -> ()
                        }
                        frame 4, 5 {
                          n3571 = local write "1 5"(TRUE ("1 5")) -> ()
                        }
                        frame 6 {
                          n3572 = local write "1 11"(TRUE ("1 11")) -> ()
                        }
                      }
                      n3573 = local write "主板2"(w5172) -> ()
                    }
                    frame "从板" {
                      n3574 = case shown="4" w5187 {
                        tunnel: [T19."从板信息" ("等级 2") T19."从板信息" ("等级 2") T19."一级故障阀值" ("等级 2") T19."二级故障阀值" ("等级 2") T19."三级故障阀值" ("等级 2") T19."快换参数" ("等级 2") T14."从板信息" ("等级 2")] -> w5186
                        frame 99, Default {
                          n3575 = local write "1 6"(TRUE ("1 6")) -> ()
                        }
                        frame 0 {
                          n3576 = local write "1 6"(TRUE ("1 6")) -> ()
                        }
                        frame 1 {
